vi "Siargo Get Data.vi"(8 "error in":errorcluster, 11 "serial master instance":refnum<class "Modbus Master.lvclass">) -> (0 "error out":errorcluster, 2 "Siargo Control Output":T1, 3 "Modbus API out":refnum<class "Modbus Master.lvclass">)   [LabVIEW 2020]
uses:
  Controls/Siargo Main Control.ctl
  <vilib>/NI/Modbus Library/API/Master/Modbus Master.lvclass
  C:/Program Files (x86)/National Instruments/LabVIEW 2020/vi.lib/NI/Modbus Library/API/Modbus API.lvclass
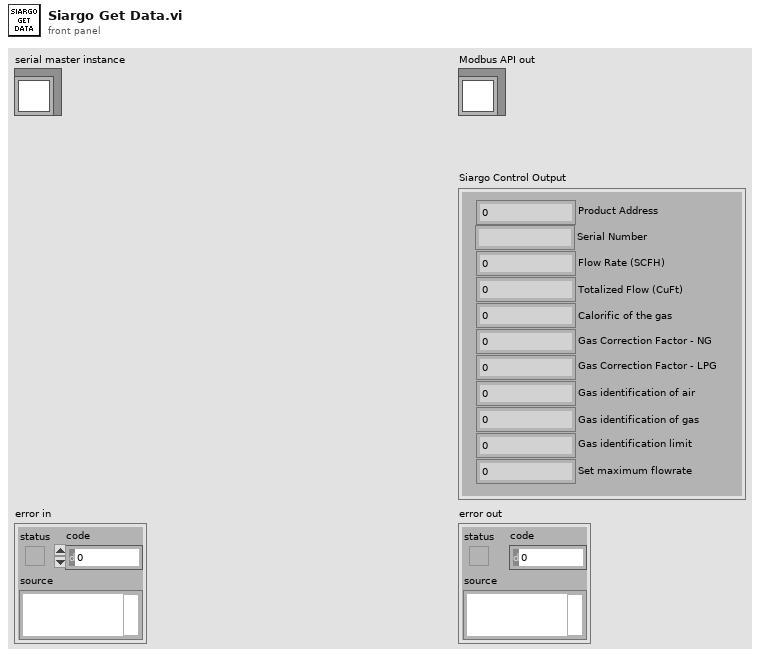
[diagram p1: front panel]
types:
  T1 = typedef "Siargo Main Control.ctl" = cluster{"Flow Rate (SCFH)":dbl, "Totalized Flow (CuFt)":dbl, "Product Address":u16, "Calorific of the gas":u16, "Gas Correction Factor - NG":u16, "Gas Correction Factor - LPG":u16, "Gas identification of air":u16, "Gas identification of gas":u16, "Gas identification limit":u16, "Set maximum flowrate":dbl, "Serial Number":string}
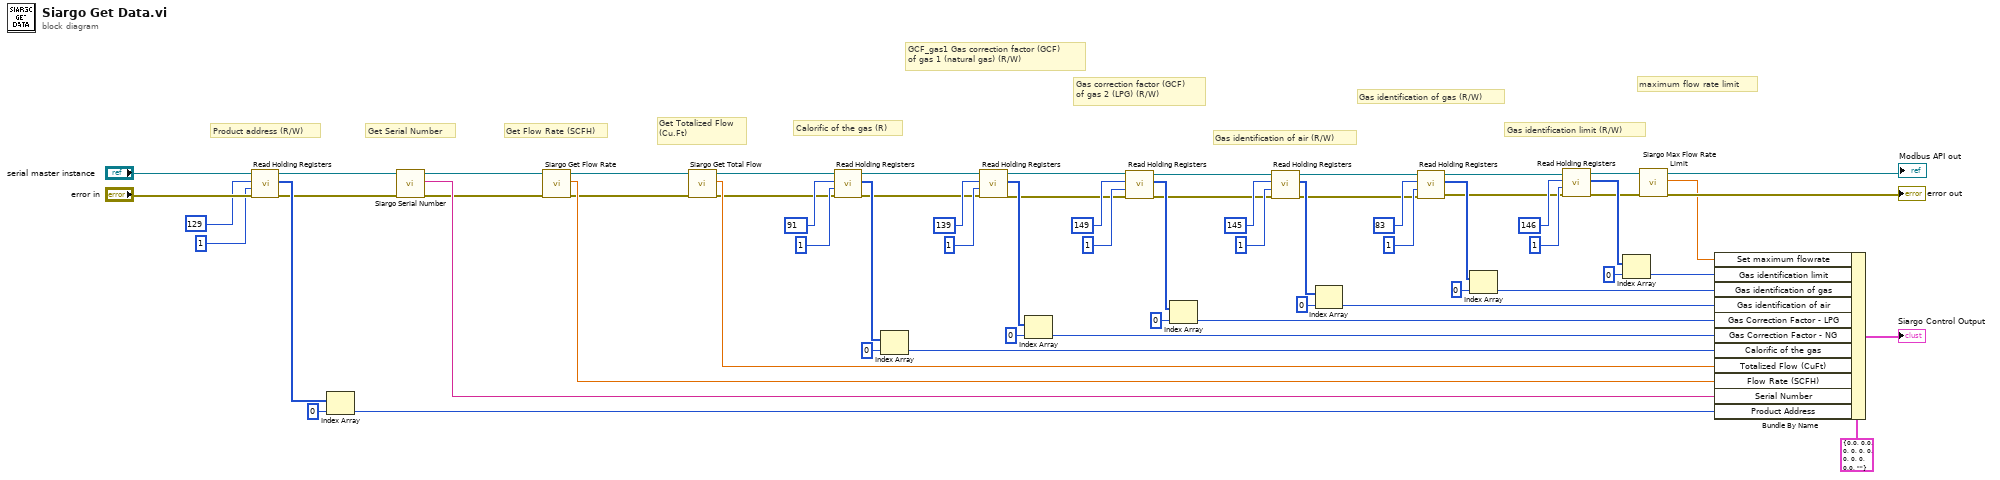
[diagram p0: block diagram]
diagram:
  # "Product address (R/W)"
  # "maximum flow rate limit"
  # "Gas identification limit (R/W)"
  # "Gas identification of gas (R/W)"
  # "Gas identification of air (R/W)"
  # "Gas correction factor (GCF)\nof gas 2 (LPG) (R/W)"
  # "Get Totalized Flow\n(Cu.Ft)"
  # "Get Flow Rate (SCFH)"
  # "Get Serial Number"
  # "GCF_gas1\tGas correction factor (GCF)\nof gas 1 (natural gas) (R/W)"
  # "Calorific of the gas (R)"
  n1 = call-dynamic "Read Holding Registers.vi"("error in"="error in", "number of inputs"=u16 1, "starting address"=u16 129, "Modbus master in"="serial master instance") -> ("error out"=w1:errorcluster, "register values"=w41:u16[], "Modbus master out"=w64:refnum<class "Modbus Master.lvclass">)  [unwired: 5 in]
  n2 = Index Array(array=w41, index=0) -> (element=w26:u16)
  n3 = call "Siargo Serial Number.vi"("error in (no error)"=w1, "Modbus API in"=w64) -> ("error out"=w2:errorcluster, "Serial Number"=w25:string, "Modbus API out"=w63:refnum<class "Modbus Master.lvclass">)  [unwired: 7 in]
  n4 = call "Siargo Get Flow Rate.vi"("error in (no error)"=w2, "Modbus API in"=w63) -> ("error out"=w3:errorcluster, "Flow Rate (SCFH)"=w24:dbl, "Modbus API out"=w62:refnum<class "Modbus Master.lvclass">)  [unwired: 7 in]
  n5 = call "Siargo Get Total Flow.vi"("error in (no error)"=w3, "Modbus API in"=w62) -> ("error out"=w4:errorcluster, "Totalized Flow (CuFt)"=w23:dbl, "Modbus API out"=w59:refnum<class "Modbus Master.lvclass">)  [unwired: 7 in]
  n6 = call-dynamic "Read Holding Registers.vi"("error in"=w4, "number of inputs"=u16 1, "starting address"=u16 91, "Modbus master in"=w59) -> ("error out"=w5:errorcluster, "register values"=w38:u16[], "Modbus master out"=w58:refnum<class "Modbus Master.lvclass">)  [unwired: 5 in]
  n7 = Index Array(array=w38, index=0) -> (element=w22:u16)
  n8 = call-dynamic "Read Holding Registers.vi"("error in"=w5, "number of inputs"=u16 1, "starting address"=u16 139, "Modbus master in"=w58) -> ("error out"=w6:errorcluster, "register values"=w28:u16[], "Modbus master out"=w53:refnum<class "Modbus Master.lvclass">)  [unwired: 5 in]
  n9 = Index Array(array=w28, index=0) -> (element=w21:u16)
  n10 = call-dynamic "Read Holding Registers.vi"("error in"=w6, "number of inputs"=u16 1, "starting address"=u16 149, "Modbus master in"=w53) -> ("error out"=w7:errorcluster, "register values"=w29:u16[], "Modbus master out"=w50:refnum<class "Modbus Master.lvclass">)  [unwired: 5 in]
  n11 = Index Array(array=w29, index=0) -> (element=w20:u16)
  n12 = call-dynamic "Read Holding Registers.vi"("error in"=w7, "number of inputs"=u16 1, "starting address"=u16 145, "Modbus master in"=w50) -> ("error out"=w8:errorcluster, "register values"=w30:u16[], "Modbus master out"=w47:refnum<class "Modbus Master.lvclass">)  [unwired: 5 in]
  n13 = Index Array(array=w30, index=0) -> (element=w19:u16)
  n14 = call-dynamic "Read Holding Registers.vi"("error in"=w8, "number of inputs"=u16 1, "starting address"=u16 83, "Modbus master in"=w47) -> ("error out"=w9:errorcluster, "register values"=w31:u16[], "Modbus master out"=w44:refnum<class "Modbus Master.lvclass">)  [unwired: 5 in]
  n15 = Index Array(array=w31, index=0) -> (element=w18:u16)
  n16 = call-dynamic "Read Holding Registers.vi"("error in"=w9, "number of inputs"=u16 1, "starting address"=u16 146, "Modbus master in"=w44) -> ("error out"=w10:errorcluster, "register values"=w32:u16[], "Modbus master out"=w43:refnum<class "Modbus Master.lvclass">)  [unwired: 5 in]
  n17 = Index Array(array=w32, index=0) -> (element=w17:u16)
  n18 = call "Siargo Max Flow Rate Limit.vi"("error in (no error)"=w10, "Modbus API in"=w43) -> ("error out"=→"error out":errorcluster, "MaxFlowRate"=w16:dbl, "Modbus API out"=→"Modbus API out":refnum<class "Modbus Master.lvclass">)  [unwired: 7 in]
  n19 = Bundle By Name(cluster=T1 {"Flow Rate (SCFH)"=0.0, "Totalized Flow (CuFt)"=0.0, "Product Address"=0, "Calorific of the gas"=0, "Gas Correction Factor - NG"=0, "Gas Correction Factor - LPG"=0, "Gas identification of air"=0, "Gas identification of gas"=0, "Gas identification limit"=0, "Set maximum flowrate"=0.0, "Serial Number"=""} ("Siargo Control Input"), "Set maximum flowrate"=w16, "Gas identification limit"=w17, "Gas identification of gas"=w18, "Gas identification of air"=w19, "Gas Correction Factor - LPG"=w20, "Gas Correction Factor - NG"=w21, "Calorific of the gas"=w22, "Totalized Flow (CuFt)"=w23, "Flow Rate (SCFH)"=w24, "Serial Number"=w25, "Product Address"=w26) -> (→"Siargo Control Output":T1)
